vi "test_AM_factor.vi"() -> ()   [LabVIEW 2013]
uses:
  <vilib>/measure/NI_MABase.lvlib
panel:
  out "Waveform Graph 2":dbl[][](graph)
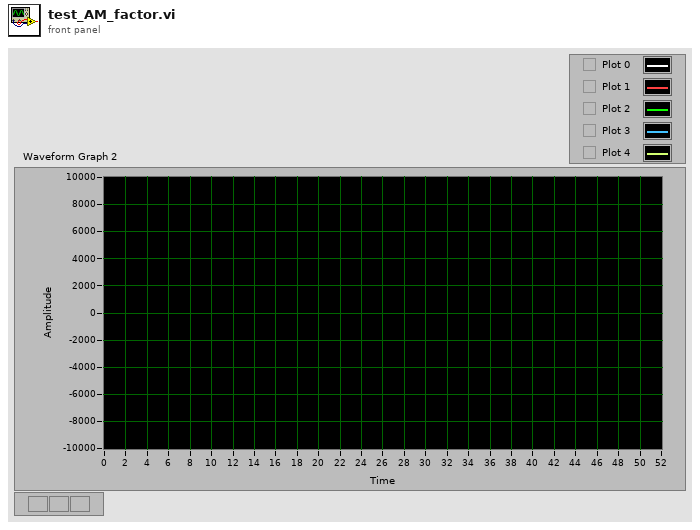
[diagram p1: front panel]
types:
  T1 = cluster{"frequency":dbl, "amplitude":dbl, "phase":dbl}[]
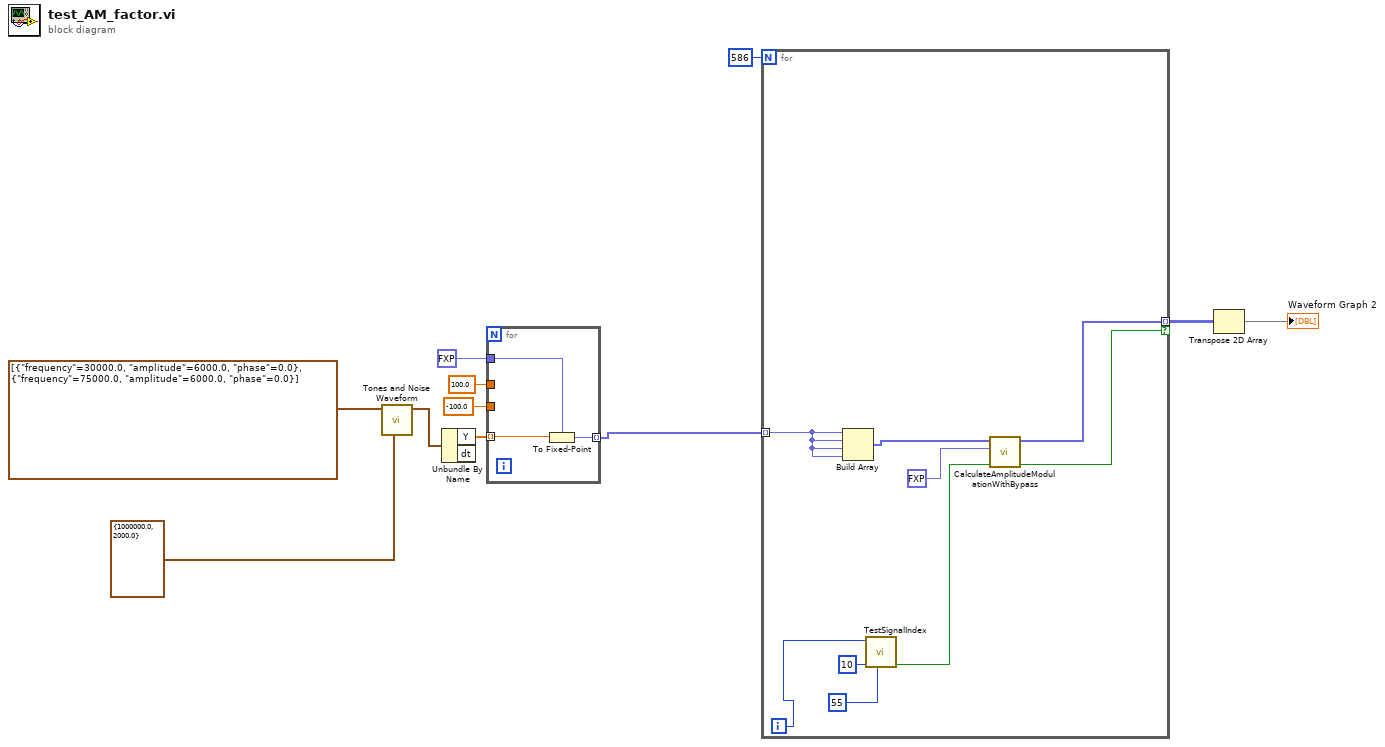
[diagram p0: block diagram]
diagram:
  n1 = call <vilib>:"Tones and Noise Waveform.vi"("sampling info"=cluster{"Fs":dbl, "#s":dbl} {"Fs"=1000000.0, "#s"=2000.0}, "tones"=T1 [{"frequency"=30000.0, "amplitude"=6000.0, "phase"=0.0}, {"frequency"=75000.0, "amplitude"=6000.0, "phase"=0.0}]) -> ("signal out"=w6:waveform(dbl))  [unwired: 8 in, 1 out]
  n2 = Unbundle By Name(w6) -> ("Y"=w7:dbl[])  [unwired: 1 out]
  n3 = for {
    tunnel: w7 -> [w12] mode=indexing
    tunnel: fxp<+/-,16,14> 0.0 ("fixed-point type") -> [w14]
    tunnel: [w13] -> w3 mode=indexing
    tunnel: 100.0 -> [_]
    tunnel: -100.0 -> [_]
    n4 = To Fixed-Point(fixed-point type=w14, number=w12) -> (fixed-point=w13:fxp<+/-,16,14>)
  }
  n5 = for {
    N: 586 -> [_]
    tunnel: [w16] -> w11 mode=indexing if=w15
    tunnel: w3 -> [w18] mode=indexing
    i -> [w21]
    n6 = Build Array(w18, w18, w18, w18) -> (w17:fxp<+/-,16,14>[])
    n7 = call "TestSignalIndex.vi"("initial delay"=55, "cycles per sample"=10, "index"=w21) -> ("valid out"=w20:bool)  [unwired: 7 in, 1 out]
    n8 = call "CalculateAmplitudeModulationWithBypass.vi"("input valid"=w20, "AM_factor"=fxp<+/-,16,2> 1.0, "Data in"=w17) -> ("output valid"=w15:bool, "Data out"=w16:fxp<+/-,16,14>[])  [unwired: 7 in]
  }
  n9 = Transpose 2D Array(2D array=w11) -> (transposed array=→"Waveform Graph 2":fxp<+/-,16,14>[][])
